vi "Init.vi"(8 "error in (no error)":errorcluster) -> (0 "error out":errorcluster, 3 "ElfHeap out":refnum<class "ElfHeap.lvclass">)   [LabVIEW 2017, in "ElfHeap.lvclass"]
uses:
  ElfHeap.lvclass
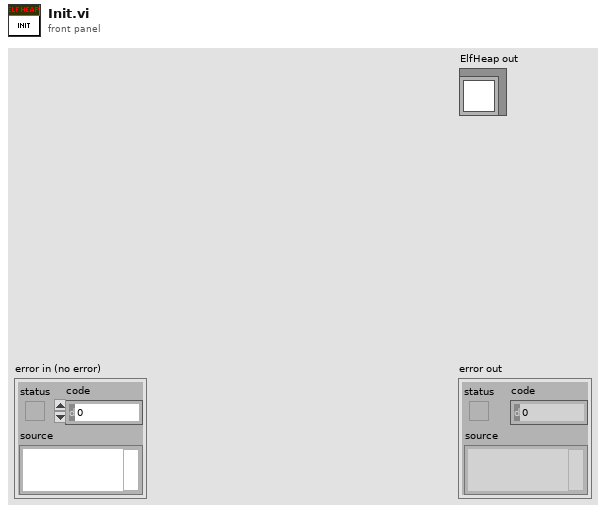
[diagram p1: front panel]
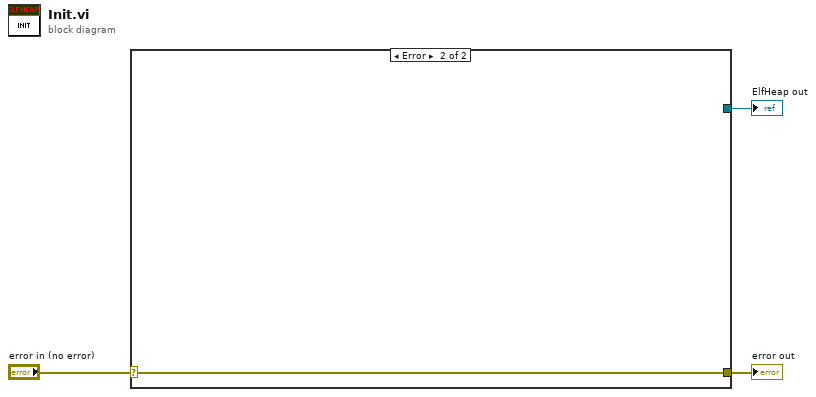
[diagram p0: block diagram]
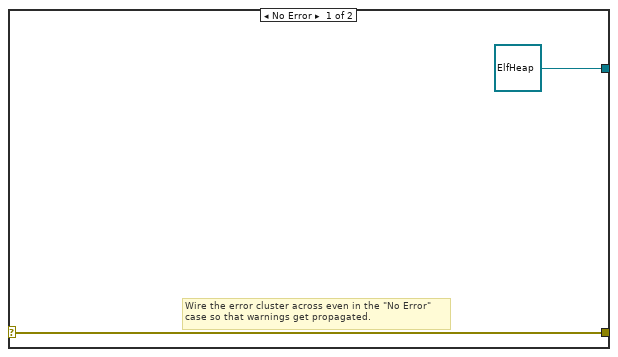
[diagram p2: hidden frame]
diagram:
  n1 = case shown="Error" "error in (no error)" {
    selector: "error in (no error)" -> [w5 w6]
    tunnel: [w5 w6] -> w2
    tunnel: [refnum<class "ElfHeap.lvclass"> refnum ("ElfHeap in") _] -> w1
    frame No Error {
      # "Wire the error cluster across even in the \"No Error\"\ncase so that warnings get propagated."
    }
    frame Error {
    }
  }
  "error out" <- w2
  "ElfHeap out" <- w1
